vi "ScanDelayMotorStatus.vi"(8 "error in (no error)":errorcluster, 9 "wait":u32=10, 11 "VISA resource name in":refnum<visa-resource-name>) -> (0 "error out":errorcluster, 2 "value":bool, 3 "VISA resource name out":refnum<visa-resource-name>)   [LabVIEW 2018]
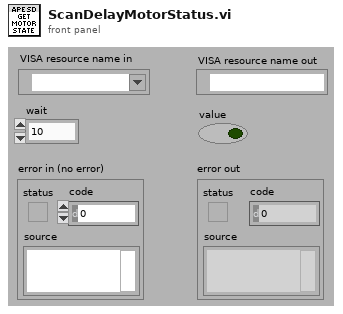
[diagram p1: front panel]
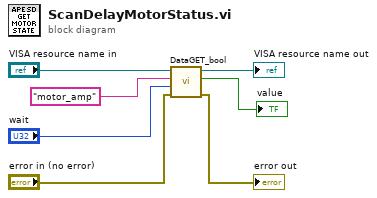
[diagram p0: block diagram]
diagram:
  n1 = call "DataGET_bool.vi"("error in"="error in (no error)", "wait"="wait", "parameter"="motor_amp", "VISA resource name"="VISA resource name in") -> ("error out"=→"error out":errorcluster, "value"=→"value":bool, "VISA resource name out"=→"VISA resource name out":refnum<visa-resource-name>)  [unwired: 4 in]
